vi "Dashboard Main.vi"() -> ()   [LabVIEW 2015]
uses:
  Common Code/Auton Command Cluster.ctl
  Common Code/Auton File Lists.ctl
  Vision/Camera Types.ctl
  Common Code/Goal Vision Packet.ctl
  <vilib>/Rock Robotics/WPI/Camera/WPI_CameraSettings Read MJPG.ctl
  <vilib>/Rock Robotics/WPI/Camera/WPI_CameraImageSize.ctl
  Common Code/Encoder Values Super Cluster.ctl
  Common Code/Encoder Values.ctl
  Common Code/Power and Diagnostic Data.ctl
  Common Code/Utilities/PDP Data.ctl
  Common Code/Utilities/PCM Data.ctl
  Common Code/IMU Data.ctl
  navX-MXP Library/COMMON/TypeDefs/Value TypeDefs/navX NAVX_CAL_STATUS.ctl
  navX-MXP Library/COMMON/TypeDefs/Value TypeDefs/navX NAVX_OP_STATUS.ctl
  Common Code/Intake Status Cluster.ctl
  Common Code/Intake Mode.ctl
  Common Code/Intake States.ctl
  Common Code/Climb Status Cluster.ctl
  Common Code/Climb Presets.ctl
  Common Code/Major Loop Times.ctl
  Common Code/Shooter State Cluster.ctl
  Common Code/Shooter State.ctl
  Common Code/Shoot Modes Enum.ctl
  Common Code/Shot Type.ctl
  Common Code/Encoder Control.ctl
  Common Code/Drivetrain Status Cluster.ctl
  Common Code/Drivetrain Modes.ctl
  Common Code/Dist Drive Status.ctl
  Common Code/Drivetrain Settings.ctl
  Common Code/Shooter Presets.ctl
  Common Code/Shot Presets.ctl
  Common Code/Intake Presets.ctl
  Common Code/Drivetrain Output Range.ctl
  Common Code/Ultrasonic Data.ctl
  Common Code/Dashboard Communication/Dashboard Control Data.ctl
  Common Code/Dashboard Drivetrain Command.ctl
  Common Code/Drivetrain Vision.ctl
  Common Code/Ball Tracking Command Cluster.ctl
  Common Code/Ball Vision Packet.ctl
  Common Code/Tracking Mode.ctl
  Common Code/IntakeEcoderControl.ctl
  Common Code/Dashboard Communication/Dashboard Display Data.ctl
  <vilib>/Rock Robotics/WPI/Dashboard/WPI_DashboardLogging Global.vi
  <vilib>/Utility/inputDevices.llb/keyboardAcquire.vi
  navX-MXP Library/navX-MXP IMU.lvlib
panel:
  in  "Logging Filename":path=path ""
  in  "stop":bool
  out "DumbDashMessage":string="111 values loaded OK"
  in  "Save":bool
  in  "Load":bool
  in  "TCP":refnum<k5>
  in  "Rec Mode":enum32{"Stop", "Record", "Playback"}(radio)
  out "Image Message":string="Timeout in Camera Communications"
  in  "Dashboard Tab":T1(tab)=enum."Shoot"
  out "Intake State":bool
  out "Right RPM":dbl(knob) scale=0.0..5000.0
  out "Left RPM":dbl(knob) scale=0.0..5000.0
  out "Mode":T2(ring)=enum."Disconnected"
  out "Shooter Mode":bool
  out "Gyro":dbl(knob) scale=0.0..360.0 scale format="%#.7g"
  out "Climb Mode":bool
  out "Intake Mode":bool
  out "Shooter State":bool
  out "Camera IP":string
  out "Robot IP":string
  out "Angle Ready?":bool
  out "RPM Ready?":bool
  out "Vision Ready?":bool
  out "Ball Loaded?":bool
  out "Intake High?":bool
  out "Shooter Ready?":bool
  out "Front Camera Display":T3(plugin-control)
  in  "Camera Mode":u16(ring)=3 items=["Camera Off", "USB Camera SW", "USB Camera HW", "IP Camera"]
  out "FPS":dbl
  out "Bandwidth (Mbps)":dbl
  out "NAVX_CAL_STATUS":T4 items=["IMU_CAL_STATE_MASK"=3, "IMU_CAL_INPROGRESS"=0, "IMU_CAL_ACCUMULATE"=1, "IMU_CAL_COMPLETE"=2, "MAG_CAL_COMPLETE"=4, "BARO_CAL_COMPLETE"=8]
  out "Auton Command Cluster":T5
  out "Auton File Lists":T6
  in  "Ultrasonic Limit":dbl
  in  "Roll Limit":dbl
  in  "Pitch Limit":dbl
  in  "Drivetrain Settings":T7={"Gyro Tolerance"=6.0, "Throttle Ramp (ms)"=250.0, "Angular rate compensation"=FALSE, "Throttle to Rate Scale"=0.0, "Rate compensation gain"=0.0, "Kv"=0.0, "Ka"=0.0, "Feed Forward P"=1.0, "Feed Forward D"=0.0, "Goal Vision PID gains"={"proportional gain (Kc)"=0.0, "integral time (Ti, min)"=0.0, "derivative time (Td, min)"=0.0}, "Goal Detection Window"=0.1} {"Goal Vision PID gains"."derivative time (Td, min)" format="%.3f"; "Goal Vision PID gains"."integral time (Ti, min)" format="%.3f"; "Goal Vision PID gains"."proportional gain (Kc)" format="%.3f"}
  out "Drivetrain Status Cluster":T8 {"2nd Gear Time" scale=0.0..135.0; "1st Gear Time" scale=0.0..135.0}
  in  "Encoder Settings":T11={"Right Tick Constant"=0.002781, "Left Tick Constant"=0.002785, "Reset?"=FALSE, "Y Dist"={"PID gains"={"proportional gain (Kc)"=0.0, "integral time (Ti, min)"=0.0, "derivative time (Td, min)"=0.0}}, "Y Stop Thresh"=0.0, "Y Stop Speed"=0.0}
  in  "Goal Output Range":cluster{"output high":dbl, "output low":dbl}
  out "Encoder Values":T12
  in  "Steer PID output":cluster{"output high":dbl, "output low":dbl}
  in  "Steer PID gains":T14
  in  "Shooter Presets":T15={"Batter Shot"={"Left Wheel RPM"=0.0, "Right Wheel RPM"=0.0, "Angle"=0.0}, "Deep Middle Shot"={"Left Wheel RPM"=0.0, "Right Wheel RPM"=0.0, "Angle"=0.0}, "Manual Shot"={"Left Wheel RPM"=700.0, "Right Wheel RPM"=700.0, "Angle"=0.0}, "Left Ticks Per Rotation"=-1378.0, "Right Ticks Per Rotation"=1388.0, "Low Bar Shot"={"Left Wheel RPM"=0.0, "Right Wheel RPM"=0.0, "Angle"=0.0}, "Shooter RPM Tolerance"=50.0, "IIR Filter Power"=0.0, "Trigger Power"=0.9, "Fire from Load Delay"=250, "Angle Pot M"=12.0, "Angle Pot B"=-0.1, "Shooter Length"=0.0, "String Pot Dist"=0.0, "Angle PID gains"={"proportional gain (Kc)"=1.0, "integral time (Ti, min)"=0.0, "derivative time (Td, min)"=0.002}, "Angle Motor Output"={"output high"=0.0, "output low"=0.0}, "Shooter Angle Tolerance"=3.0, "Vision Shoot x^2"=0.0, "Vision Shoot x"=0.0, "Dist from Axis Cam to Pivot"=23.375, "High Goal Center Height"=97.0, "Feed Forward Max Accel"=0.0, "Feed Forward Kv"=0.005, "Backwards Trigger"=-0.4, "Shot Finish Delay (ms)"=250.0, "Angle Max Current"=40.0, "Angle Current Trip Time"=500.0, "Shooter Intake Angle"=0.0, "Vision Shoot c"=0.0, "Reset?"=FALSE, "Servo Release Delay"=0.0, "Servo Idle Angle"=108, "Servo Hold Angle"=55, "Angle Pot x^2"=0.0, "Angle Pot x"=0.0, "Angle Pot c"=0.0, "Ignore Angle?"=FALSE} {"Angle Motor Output"."output low" format="%.2f"; "Angle Motor Output"."output high" format="%.2f"}
  out "Shooter State Cluster":T17 {"Trigger Output" scale=-1.0..1.0; "Angle Motor Output" scale=-1.0..1.0; "Right RPM" scale=0.0..5000.0; "Left RPM" scale=0.0..5000.0}
  in  "Intake Presets":T21={"Intake Speed"=0.8, "Outake Speed"=-0.8, "Low Height"=0.0, "Half Height"=55.0, "Full Height"=90.0, "Angle Speed"=0.0, "Fast Angle"=0.0, "Encoder Scale"=0.001478, "Load Height"=30.0, "Output Range"={"output high"=0.0, "output low"=0.0}, "Rotation Power Max/Min"=0.5, "MaxCurrent"=40.0, "Intake Trip Time"=500.0, "Idle Height"=40.0, "Max Height"=90.0, "Reset Encoders?"=FALSE, "PID gains"={"proportional gain (Kc)"=1.0, "integral time (Ti, min)"=0.0, "derivative time (Td, min)"=0.0}} {"Max Height" format="%#_7g"; "Idle Height" format="%#_7g"; "Intake Trip Time" format="%#_7g"; "MaxCurrent" format="%#_7g"; "Rotation Power Max/Min" format="%#_7g"; "Load Height" format="%#_7g"; "Encoder Scale" format="%#_7g"; "Fast Angle" format="%#_7g"; "Angle Speed" format="%#_7g"; "Full Height" format="%#_7g"; "Half Height" format="%#_7g"; "Low Height" format="%#_7g"; "Outake Speed" format="%#_7g"; "Intake Speed" format="%#_7g"}
  out "Intake Status Cluster":T23
  in  "Climb Presets":T26
  out "Climb Status Cluster":T27
  out "IMU Data":T28 {"NAVX_OP_STATUS" items=["INITIALIZING", "SELFTEST_IN_PROGRESS", "ERROR", "IMU_AUTOCAL_IN_PROGRESS", "NORMAL"]; "NAVX_CAL_STATUS" items=["IMU_CAL_STATE_MASK"=3, "IMU_CAL_INPROGRESS"=0, "IMU_CAL_ACCUMULATE"=1, "IMU_CAL_COMPLETE"=2, "MAG_CAL_COMPLETE"=4, "BARO_CAL_COMPLETE"=8]}
  out "Gyro 2":dbl(knob) scale=0.0..360.0 scale format="%#.7g"
  out "Ultrasonic Data":T30
  out "Camera Display 2":T3(plugin-control)
  in  "Aspect Fudge Factor":dbl=1.0
  in  "Score Threshold 2":dbl=75.0 format="%#_13g"
  out "Goal Display":T3(plugin-control)
  out "Found Targets":T31(array[cluster]) {"Normalized Rect"."Numeric 5" format="%#_2g"; "Normalized Rect"."Numeric 3" format="%#_2g"; "Normalized Rect"."Numeric 2" format="%#_2g"; "Normalized Rect"."Numeric" format="%#_2g"}
  in  "Camera Type":T32=enum."1011"
  out "Goal Vision Packet":T33
  in  "Camera Settings 2":T34={"fps"=30, "compression"=30, "Image Size"=enum."320x240"}
  in  "File number":i32
  in  "Use Goal File?":bool
  in  "Color Components":T36={"Hue"={110.0, 142.0}, "Sat"={138.0, 255.0}, "Val"={139.0, 198.0}} {"Val" scale=0.0..255.0; "Sat" scale=0.0..255.0; "Hue" scale=0.0..255.0 scale format="%#_3g"}
  out "Goal Active?":bool
  out "Power and Diagnostic Data":T37
  out "Control Info":T40
  out "Status Info":T41
  out "DS TCP":T42
  out "Robot Metrics":T43
  out "Loop Times":T44
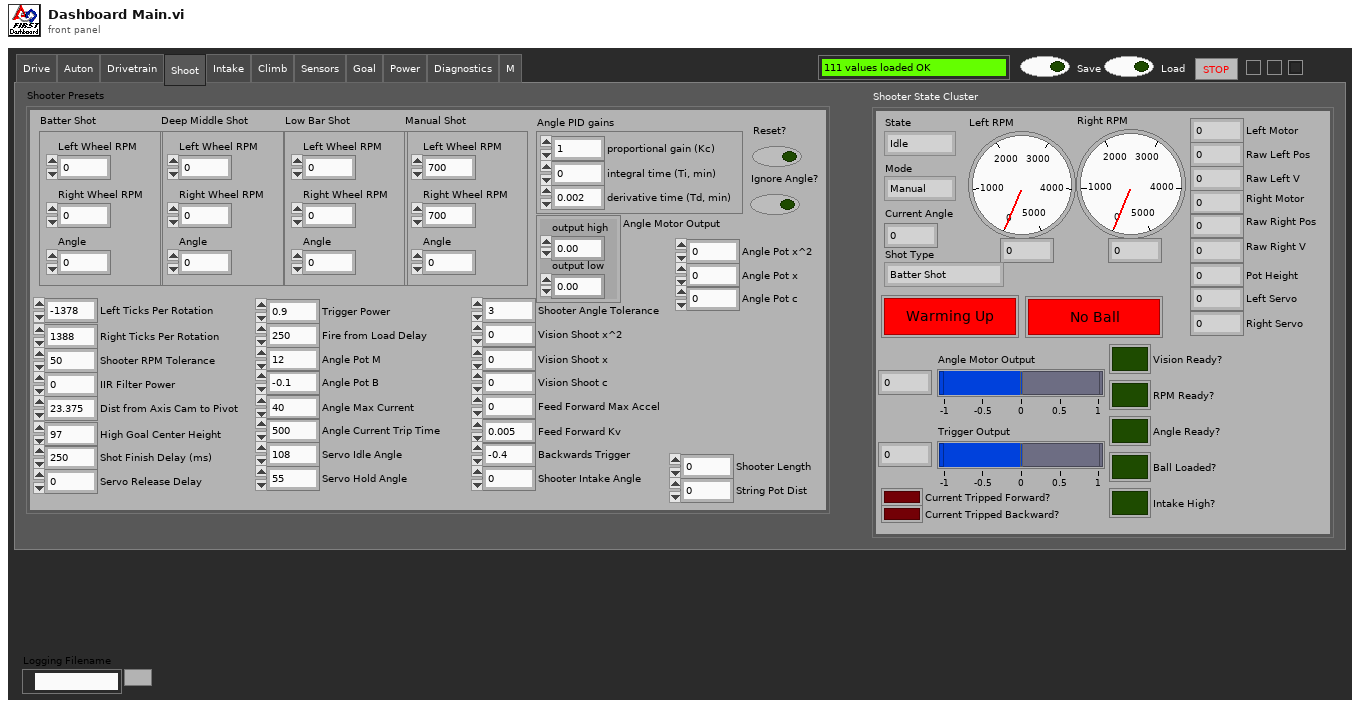
[diagram p1: front panel]
types:
  T1 = enum32{"Drive", "Auton", "Drivetrain", "Shoot", "Intake", "Climb", "Sensors", "Goal", "Power", "Diagnostics", "M"}
  T2 = enum8{"Tele-Op Disabled", "Tele-Op Enabled", "Auto Disabled", "Auto Enabled", "Test Disabled", "Test Enabled", "Disconnected", "No Code", "E-Stop"}
  T3 = typedef "IMAQ Image.ctl" = refnum<image>
  T4 = typedef "navX-MXP IMU.lvlib/navX NAVX_CAL_STATUS.ctl" = u8
  T5 = typedef "Auton Command Cluster.ctl" = cluster{"Command ID":i32, "maxTime":dbl, "Y Distance":dbl, "Heading":dbl, "Throttle":dbl, "Async":dbl, "Velocity":dbl, "Acceleration":dbl, "To":dbl, "Condition":dbl, "Shot Type":dbl, "Left RPM":dbl, "Override RPM":i32, "Override Angle":i32, "Right RPM":dbl, "Angle":dbl, "Intake Mode":i32, "Intake Cmd":i32, "Intake O":i32, "Eject O":i32, "Angle O":i32, "Arm O":i32, "Intake Speed":dbl, "Eject Speed":dbl, "Arm Angle":dbl, "Arm Speed":dbl, "Intake?":i32, "Eject?":i32}
  T6 = typedef "Auton File Lists.ctl" = cluster{"Current Queue":string, "General Scripts":string, "Defense Scripts":string, "Movement Scripts":string}
  T7 = typedef "Drivetrain Settings.ctl" = cluster{"Gyro Tolerance":dbl, "Throttle Ramp (ms)":dbl, "Angular rate compensation":bool, "Throttle to Rate Scale":dbl, "Rate compensation gain":dbl, "Kv":dbl, "Ka":dbl, "Feed Forward P":dbl, "Feed Forward D":dbl, "Goal Vision PID gains":cluster{"proportional gain (Kc)":dbl, "integral time (Ti, min)":dbl, "derivative time (Td, min)":dbl}, "Goal Detection Window":dbl}
  T8 = typedef "Drivetrain Status Cluster.ctl" = cluster{"Modes":T9, "Y (Throttle)":dbl, "X (Steer)":dbl, "Gyro In Range?":bool, "Distance Drive Finished?":bool, "Stop Eject Lockout":bool, "Dist Drive Status":T10, "Y Target":dbl, "Heading Target":dbl, "Vision Target Aligned?":bool, "Gear":dbl, "1st Gear Time":dbl, "2nd Gear Time":dbl, "1st Gear Shifts":dbl, "2nd Gear Shifts":dbl}
  T9 = typedef "Drivetrain Modes.ctl" = enum16{"Climb", "Manual", "Ball Vision Targeting", "Goal Vision Targeting", "PID Distance Drive", "Hybrid"}
  T10 = typedef "Dist Drive Status.ctl" = cluster{"Y In Range":bool, "X In Range":bool, "Gyro In Range":bool, "Y Dist":dbl, "X Dist":dbl, "Gyro":dbl}
  T11 = typedef "Encoder Control.ctl" = cluster{"Right Tick Constant":dbl, "Left Tick Constant":dbl, "Reset?":bool, "Y Dist":cluster{"PID gains":cluster{"proportional gain (Kc)":dbl, "integral time (Ti, min)":dbl, "derivative time (Td, min)":dbl}}, "Y Stop Thresh":dbl, "Y Stop Speed":dbl}
  T12 = typedef "Encoder Values Super Cluster.ctl" = cluster{"Left Encoder":T13, "Right Encoder":T13}
  T13 = typedef "Encoder Values.ctl" = cluster{"Distance":dbl, "Speed":dbl, "Ticks":dbl}
  T14 = cluster{"proportional gain (Kc)":dbl, "integral time (Ti, min)":dbl, "derivative time (Td, min)":dbl}
  T15 = typedef "Shooter Presets.ctl" = cluster{"Batter Shot":T16, "Deep Middle Shot":T16, "Manual Shot":T16, "Left Ticks Per Rotation":dbl, "Right Ticks Per Rotation":dbl, "Low Bar Shot":T16, "Shooter RPM Tolerance":dbl, "IIR Filter Power":dbl, "Trigger Power":dbl, "Fire from Load Delay":i32, "Angle Pot M":dbl, "Angle Pot B":dbl, "Shooter Length":dbl, "String Pot Dist":dbl, "Angle PID gains":cluster{"proportional gain (Kc)":dbl, "integral time (Ti, min)":dbl, "derivative time (Td, min)":dbl}, "Angle Motor Output":cluster{"output high":dbl, "output low":dbl}, "Shooter Angle Tolerance":dbl, "Vision Shoot x^2":dbl, "Vision Shoot x":dbl, "Dist from Axis Cam to Pivot":dbl, "High Goal Center Height":dbl, "Feed Forward Max Accel":dbl, "Feed Forward Kv":dbl, "Backwards Trigger":dbl, "Shot Finish Delay (ms)":dbl, "Angle Max Current":dbl, "Angle Current Trip Time":dbl, "Shooter Intake Angle":dbl, "Vision Shoot c":dbl, "Reset?":bool, "Servo Release Delay":dbl, "Servo Idle Angle":i32, "Servo Hold Angle":i32, "Angle Pot x^2":dbl, "Angle Pot x":dbl, "Angle Pot c":dbl, "Ignore Angle?":bool}
  T16 = typedef "Shot Presets.ctl" = cluster{"Left Wheel RPM":dbl, "Right Wheel RPM":dbl, "Angle":dbl}
  T17 = typedef "Shooter State Cluster.ctl" = cluster{"State":T18, "Left RPM":dbl, "Right RPM":dbl, "Shooter Ready?":bool, "Ball Loaded?":bool, "Current Angle":dbl, "Angle Motor Output":dbl, "Trigger Output":dbl, "Angle Ready?":bool, "RPM Ready?":bool, "Vision Ready?":bool, "Ball Loaded?":bool, "Mode":T19, "Shot Type":T20, "Pot Height":dbl, "Current Tripped Forward?":bool, "Current Tripped Backward?":bool, "Left Motor":dbl, "Right Motor":dbl, "Intake High?":bool, "Raw Left Pos":dbl, "Raw Right Pos":dbl, "Raw Left V":dbl, "Raw Right V":dbl, "Right Servo":i32, "Left Servo":i32}
  T18 = typedef "Shooter State.ctl" = enum16{"Idle", "Warmup", "Shooter Ready", "Shoot"}
  T19 = typedef "Shoot Modes Enum.ctl" = enum16{"Manual", "Safe", "Auto"}
  T20 = typedef "Shot Type.ctl" = enum16{"Batter Shot", "Corner Shot", "Curve Shot", "Vision Shot", "Deep Middle Shot"}
  T21 = typedef "Intake Presets.ctl" = cluster{"Intake Speed":dbl, "Outake Speed":dbl, "Low Height":dbl, "Half Height":dbl, "Full Height":dbl, "Angle Speed":dbl, "Fast Angle":dbl, "Encoder Scale":dbl, "Load Height":dbl, "Output Range":T22, "Rotation Power Max/Min":dbl, "MaxCurrent":dbl, "Intake Trip Time":dbl, "Idle Height":dbl, "Max Height":dbl, "Reset Encoders?":bool, "PID gains":cluster{"proportional gain (Kc)":dbl, "integral time (Ti, min)":dbl, "derivative time (Td, min)":dbl}}
  T22 = typedef "Drivetrain Output Range.ctl" = cluster{"output high":dbl, "output low":dbl}
  T23 = typedef "Intake Status Cluster.ctl" = cluster{"Roller Power":dbl, "Angle Power":dbl, "Intake Mode":T24, "Intake States":T25, "Rollers Active?":bool, "Current Height":dbl, "Target Height":dbl, "Encoder Raw Position":dbl, "Forward Tripped?":bool, "Backward Tripped?":bool, "Override IR?":bool}
  T24 = typedef "Intake Mode.ctl" = enum16{"Safe", "Auto", "Manual"}
  T25 = typedef "Intake States.ctl" = enum16{"Idle", "Set roller speed", "Move to angle"}
  T26 = typedef "Climb Presets.ctl" = cluster{"Pull Power":dbl, "Unpin Power":dbl, "Time to Hold":dbl}
  T27 = typedef "Climb Status Cluster.ctl" = cluster{"Pull Power":dbl, "Unpin Power":dbl, "PTO Engaged?":bool, "Pull Height":dbl}
  T28 = typedef "IMU Data.ctl" = cluster{"Pitch":sgl, "Roll":sgl, "Yaw":sgl, "Data Valid?":bool, "Temp":sgl, "MOVING":bool, "YAW_STABLE":bool, "Accel X":sgl, "Accel Y":sgl, "Accel Z":sgl, "Accel Magnitude":sgl, "Pitch Rate":sgl, "Roll Rate":sgl, "Yaw Rate":sgl, "NavX Opened?":bool, "NAVX_CAL_STATUS":T4, "NAVX_OP_STATUS":T29}
  T29 = typedef "navX-MXP IMU.lvlib/navX NAVX_OP_STATUS.ctl" = u8
  T30 = typedef "Ultrasonic Data.ctl" = cluster{"Left Ultrasonic":dbl, "Right Ultrasonic":dbl}
  T31 = cluster{"Distance (ft)":dbl, "Center":cluster{dbl, dbl}, "Normalized Rect":cluster{"Numeric":dbl, "Numeric 2":dbl, "Numeric 3":dbl, "Numeric 5":dbl}}[]
  T32 = typedef "Camera Types.ctl" = enum16{"206", "1011", "1013", "MS HD3000 square", "MS HD3000 640x480"}
  T33 = typedef "Goal Vision Packet.ctl" = cluster{"Distance":dbl, "Center X":dbl, "Center Y":dbl, "Found Target?":bool}
  T34 = typedef "WPI_CameraSettings Read MJPG.ctl" = cluster{"fps":i32, "compression":i32, "Image Size":T35}
  T35 = typedef "WPI_CameraImageSize.ctl" = enum16{"640x480", "320x240", "160x120", "Custom"}
  T36 = cluster{"Hue":cluster{dbl, dbl}, "Sat":cluster{dbl, dbl}, "Val":cluster{dbl, dbl}}
  T37 = typedef "Power and Diagnostic Data.ctl" = cluster{"PDP Data":T38, "PCM Data":T39, "roboRIO input voltage (V)":dbl, "roboRIO input current (A)":dbl, "3.3V Rail Short":bool, "5 V Rail Short":bool, "6 V Rail Short":bool, "roboRIO Brownout":bool, "Outputs Enabled?":bool}
  T38 = typedef "PDP Data.ctl" = cluster{"Battery Voltage":sgl, "Temperature (degrees C)":sgl, "Internal Battery R (Ohms)":sgl, "Energy (J)":sgl, "Power (W)":sgl, "Total Current (A)":sgl, "Battery Voltage Fault":bool, "Temperature Fault":bool, "Hardware Fault":bool, "Currents":cluster{"[0]":sgl, "[1]":sgl, "[2]":sgl, "[3]":sgl, "[4]":sgl, "[5]":sgl, "[6]":sgl, "[7]":sgl, "[8]":sgl, "[9]":sgl, "[10]":sgl, "[11]":sgl, "[12]":sgl, "[13]":sgl, "[14]":sgl, "[15]":sgl}, "Current Faults":cluster{"[0]":bool, "[1]":bool, "[2]":bool, "[3]":bool, "[4]":bool, "[5]":bool, "[6]":bool, "[7]":bool, "[8]":bool, "[9]":bool, "[10]":bool, "[11]":bool, "[12]":bool, "[13]":bool, "[14]":bool, "[15]":bool}}
  T39 = typedef "PCM Data.ctl" = cluster{"Compressor Fault":bool, "Solenoid Fault":bool, "Compressor Enabled":bool, "Hardware Fault":bool, "Compressor Current":dbl}
  T40 = cluster{"Control Bits":cluster{"TestMode":bool, "Autonomous":bool, "Enabled":bool, "FMS Present":bool, bool, bool, bool, "E-Stop":bool}, "Team Station ":u8, "Countdown":sgl, "Joystick Values":cluster{"Axes":dbl[], "Buttons":bool[], "POVs":i16[]}[]}
  T41 = cluster{"Status bits":cluster{"Test Mode":bool, "Autonomous":bool, "Enabled":bool, "Code Start":bool, "Brownout":bool, "Reserved 2":bool, "Reserved 3":bool, "E-Stop":bool}, "Code Trace":cluster{"Disabled":bool, "TeleOp":bool, "Auto":bool, "Test":bool}, "Controller Type":enum16{"unknown", "cRIO", "roboRio"}, "Code?":enum16{"unknown", "noCode", "code"}, "Battery V":dbl}
  T42 = cluster{"Error Strings":string, "Disable Counts":cluster{u16, u16}, "Rail Faults":cluster{u16, u16, u16}, "Robot IP":string, "DB Mode":u8, "Event Info":cluster{"Name":string, "Type":u8, "Number":u16, "Replay":u8}, "Camera Addr":string}
  T43 = cluster{"Storage":cluster{"Disk Free":u64, "RAM Block":u32, "RAM free":u32}, "CPU Utilization":cluster{"CPU % ISR":sgl, "CPU % Time Crit":sgl, "CPU % Timed Str":sgl, "CPU % High":sgl, "CPU % Above":sgl, "CPU % Normal":sgl, "CPU % Low":sgl}, "CAN":cluster{"% Bus Utilization":sgl, "Bus Off Cnt":u32, "TX_FIFO Full Cnt":u32, "Receive Error Cnt":u8, "Transmit Error Cnt":u8}, "HID":cluster{"HID Outputs":u32, "Rumble Low":u16, "Rumble High":u16}[]}
  T44 = typedef "Major Loop Times.ctl" = cluster{"DT Loop Timer":u32, "Shooter Loop Timer":u32, "Intake Loop Timer":u32, "US Loop Timer":u32, "Auton File Loop Timer":u32}
  T45 = typedef "Image Type" = u32
  T46 = cluster{cluster{dbl, dbl}, cluster{dbl, dbl}, cluster{dbl, dbl}}
  T47 = cluster{"Score":sgl, "Fitted Circle":cluster{"Center":cluster{"X":sgl, "Y":sgl}, "Radius":dbl, "Circle Rect":cluster{"L":sgl, "T":sgl, "R":sgl, "B":sgl}, "Roundness":dbl, "SNR (dB)":dbl}, "Search Rect":cluster{"L":sgl, "T":sgl, "R":sgl, "B":sgl}, "Details":cluster{"Edge":sgl, "Area":sgl, "Circ":sgl, "Diam":sgl}}[]
  T48 = typedef "Ball Tracking Command Cluster.ctl" = cluster{"Distance to Ball":dbl, "Desired Angle":dbl, "Command":enum16{"Turn to Ball", "Turn to Angle", "Get Distance"}, "Pixels from Center":dbl}
  T49 = typedef "Tracking Mode.ctl" = enum16{"Turn to Ball", "Turn to Angle"}
  T50 = enum16{"Turn to Ball", "Turn to Angle", "Get Distance"}
  T51 = typedef "NI_LVConfig.lvlib/Config Data RefNum.ctl" = refnum<k1>
  T52 = cluster{"Bounding box":cluster{"left":dbl, "top":dbl, "right":dbl, "bottom":dbl}, "Aspect Ratio":dbl, "Area to CH":dbl, "X Mask":dbl, "Y Mask":dbl, "Moment":dbl}[]
  T53 = cluster{"Distance (ft)":dbl, "Center":cluster{dbl, dbl}, "Normalized Rect":cluster{"Numeric":dbl, "Numeric 2":dbl, "Numeric 3":dbl, "Numeric 5":dbl}}
  T54 = typedef "Dashboard Display Data.ctl" = cluster{"Auton Command Cluster":T5, "Auton File Lists":T6, "Drivetrain Status Cluster":T8, "Encoder Values":T12, "IMU Data":T28, "Power and Diagnostic Data":T37, "Gyro":dbl, "Shooter State Cluster":T17, "Intake Status Cluster":T23, "Ultrasonic Data":T30, "Climb Status Cluster":T27, "Loop Times":T44}
  T55 = typedef "Dashboard Control Data.ctl" = cluster{"Shooter Presets":T15, "Encoder Control":T11, "Steer PID output":cluster{"output high":dbl, "output low":dbl}, " Steer PID gains":cluster{"proportional gain (Kc)":dbl, "integral time (Ti, min)":dbl, "derivative time (Td, min)":dbl}, "Drivetrain Settings":T7, "Vision Packet":T33, "Dashboard Drivetrain Command":T56, "Info/Command Cluster":T48, "Ball Vision Packet":T58, "Intake Presets":T21, "Intake Encoder Control":T59, "Climb Presets":T26, "Ultrasonic Limit":dbl, "Roll Limit":dbl, "Pitch Limit":dbl, "Goal Output Range":cluster{"output high":dbl, "output low":dbl}}
  T56 = typedef "Dashboard Drivetrain Command.ctl" = cluster{"Drivetrain Vision":T57}
  T57 = typedef "Drivetrain Vision.ctl" = cluster{"Goal Window":dbl, "Ball Window":dbl}
  T58 = typedef "Ball Vision Packet.ctl" = cluster{"Ball Detected?":bool, "Distance to Ball":dbl, "Desired Angle":dbl, "Pixels from Center":dbl, "Tracking mode":T49}
  T59 = typedef "IntakeEcoderControl.ctl" = cluster{"Arm Tick Constant":dbl, "Reset?":bool, "Y Dist":cluster{"PID gains":cluster{"proportional gain (Kc)":dbl, "integral time (Ti, min)":dbl, "derivative time (Td, min)":dbl}}, "Y Stop Thresh":dbl, "Y Stop Speed":dbl}
  T60 = cluster{"Image Size":bool, "Image Type":bool, "Pixel Value":bool, "ROI Information":bool, "Zoom Factor":bool}
  T61 = enum16{"0", "1", "2", "3", "4", "5", "6", "7", "8", "9", "A", "B", "C", "D", "E", "F", "G", "H", "I", "J", "K", "L", "M", "N", "O", "P", "Q", "R", "S", "T", "U", "V", "W", "X", "Y", "Z", "F1", "F2", "F3", "F4", "F5", "F6", "F7", "F8", "F9", "F10", "F11", "F12", "F13", "F14", "F15", "ADD", "BACK", "BACKSLASH", "CAPITAL", "COMMA", "DECIMAL", "DELETE", "DIVIDE", "DOWN", "END", "EQUALS", "ESCAPE", "GRAVE (`)", "HOME", "INSERT", "LBRACKET", "LCONTROL", "LEFT", "L ALT", "LSHIFT", "LWIN", "MINUS", "MULTIPLY", "NEXT", "NUMLOCK", "NUMPAD_0", "NUMPAD_1", "NUMPAD_2", "NUMPAD_3", "NUMPAD_4", "NUMPAD_5", "NUMPAD_6", "NUMPAD_7", "NUMPAD_8", "NUMPAD_9", "PAUSE", "PERIOD", "PRIOR (PG UP)", "RBRACKET", "RCONTROL", "RETURN", "RIGHT", "R ALT", "RSHIFT", "RWIN", "SCROLL", "SEMICOLON", "SLASH", "SPACE", "SUBTRACT", "TAB", "UP", "ENTER (num pad)", "' (quote)"}[]
  T62 = typedef "DumbDash Control.ctl" = cluster{"Name":string, "Ref":refnum<vi>, "Type":T63}
  T63 = typedef "DumbDash Control Type.ctl" = enum16{"Invalid", "Number", "Boolean", "String"}
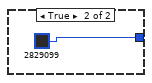
[diagram p2: hidden frame]
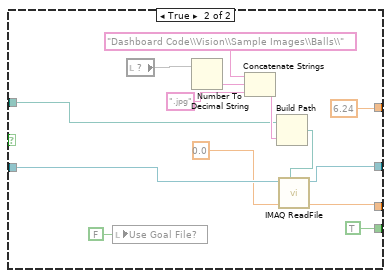
[diagram p3: hidden frame]
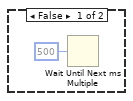
[diagram p4: hidden frame]
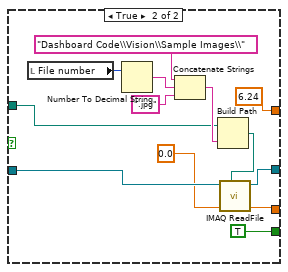
[diagram p6: hidden frame]
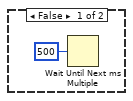
[diagram p7: hidden frame]
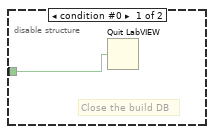
[diagram p9: hidden frame]
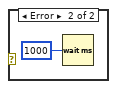
[diagram p12: hidden frame]
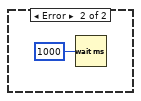
[diagram p13: hidden frame]
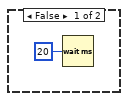
[diagram p14: hidden frame]
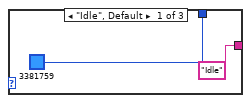
[diagram p15: hidden frame]
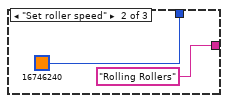
[diagram p16: hidden frame]
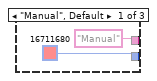
[diagram p17: hidden frame]
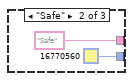
[diagram p18: hidden frame]
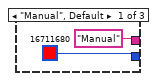
[diagram p20: hidden frame]
diagram:
  w3 = T45 0 items=["Grayscale (U8)", "Grayscale (I16)", "Grayscale (SGL)", "Complex (CSG)", "RGB (U32)", "HSL (U32)", "RGB (U64)", "Grayscale (U16)"] ("Image Type")
  w8 = T45 4 items=["Grayscale (U8)", "Grayscale (I16)", "Grayscale (SGL)", "Complex (CSG)", "RGB (U32)", "HSL (U32)", "RGB (U64)", "Grayscale (U16)"] ("Image Type")
  w11 = enum16{"Stop", "Record", "Playback"}."Stop"
  w17 = 1340
  w18 = 500
  w22 = enum32{"Stop", "Record", "Playback"}."Stop" ("Rec Mode")
  (unwired) "This VI has seven parallel loops for different tasks and a bit of initialization code that runs just once.\n\nTypical dashboard extensions only need to edit the panel. Adding new indicators or controls simply involves placing them on the panel in the Operations tab and naming them the same as the SmartDashboard variable on the robot\n\nIf the display needs to process the data before display, loop one is an example of doing that for the joysticks and motors.\n\nIf you want customize the video display or perform processing on it, loop two is where that takes place.\n\nOther loops should not need to be modified. They are pretty standard, and document the task they perform."  # Documentation
  # "Command Param Info"
  # "Started one, Unique ID holds\nresponse"
  # "Loop 7. Wait for DS connections"
  # "Basic debug and auto controls: Their data names are fixed, but\nthe displayed name, called a caption, can be changed directly or in\nrobot code such as shown in Begin."
  # "Controls for Test Mode, Camera Settings, etc."
  # "Additional UI Initialization"
  # "Loop 6. Animation for background of window during playback and record"
  # "Fires each time robot IP\nchanges, simulator does this"
  # "Fires each time window\ndocking changes."
  # "Collects all controls and indicators\nin the Basic and Custom tab.\nIf you need to bind additional controls,\nadd their references. You can extend the\nenum constant or use an integer."
  # "The remaining code below this line typically doesn't need to be modified."
  # "Loop 4. Process UI events related to test mode, checklist, and camera settings"
  # "Terminals of controls and indicators that are bound to the smart dashboard by name.\nYou can place the terminals anywhere you like and even read data from them.\nYou bind controls by adding the control reference to the array on the left. The subVI will\ndo this for the contents of a tab, and you can do it for individual items too, as shown with\nthe LED. To create get the reference, right-click and Create>>Reference."
  # "Loop 5. Adjusts placement onscreen, hides the titlebar, etc."
  # "Loop 1. Receive various data streams from Driver Station, update joystick, motors, and more complex displays that don't easily bind to variables."
  n1 = control-ref of="Rec Mode"() -> ()  [unwired: 1 out]
  n2 = control-ref of="Dashboard Tab"() -> ()  [unwired: 1 out]
  n3 = Obtain Notifier(name (unnamed)="Robot IP Update", notification data type="IP Addr" ("name (unnamed)")) -> (notifier out=w16:refnum<notifier>)  [unwired: 2 in, 2 out]
  n4 = property class="VI" props=["Front Panel.Closeable"]() -> (reference out=w21:refnum<vi>)  [unwired: 2 in, 2 out]
  n5 = Obtain Notifier(name (unnamed)="Window Mode", notification data type=TRUE) -> (notifier out=w20:refnum<notifier>)  [unwired: 2 in, 2 out]
  n6 = disable-structure shown="Disabled" {
    frame Disabled {
      w41 = T45 0 items=["Grayscale (U8)", "Grayscale (I16)", "Grayscale (SGL)", "Complex (CSG)", "RGB (U32)", "HSL (U32)", "RGB (U64)", "Grayscale (U16)"] ("Image Type")
      w43 = T45 4 items=["Grayscale (U8)", "Grayscale (I16)", "Grayscale (SGL)", "Complex (CSG)", "RGB (U32)", "HSL (U32)", "RGB (U64)", "Grayscale (U16)"] ("Image Type")
      n7 = call <vilib>:"Application Directory.vi"() -> ("Application Directory"=w40:path)
      n8 = call "IMAQ Create"("Image Name"="Ball Detection", "Image Type"=w43) -> ("New Image"=w39:T3, "error out"=w38:errorcluster)  [unwired: 3 in]
      n9 = call "IMAQ Create"("Image Name"="Ball Mask", "Image Type"=w41) -> ("New Image"=w37:T3, "error out"=w36:errorcluster)  [unwired: 3 in]
      n10 = while {
        tunnel: w38 -> [_]
        tunnel: w37 -> [w48]
        tunnel: w36 -> [_]
        tunnel: w39 -> [w52]
        tunnel: w40 -> [w53]
        stop <- FALSE stop-if-true
        n11 = case shown="False" w47 {
          tunnel: [w60 TRUE ("Active")] -> w50
          tunnel: w52 -> [w61 w75]
          tunnel: [w59 w74] -> w49
          tunnel: w53 -> [_ w70]
          tunnel: [w57 6.24 ("Bandwidth (Mbps)")] -> w46
          tunnel: [w58 0.0 ("FPS")] -> w51
          frame False {
            n12 = local read "Rec Mode"() -> (w62:enum32{"Stop", "Record", "Playback"})
            n13 = call "624WPI_CameraRead MJPG for Dashboard.vi"("Rec Mode"=w62, "Camera IP"="10.6.24.23", "Refnum in"=w61) -> ("Active"=w60:bool, "Refnum out"=w59:T3, "FPS"=w58:dbl, "Bandwidth (Mbps)"=w57:dbl, "Camera Settings"=w54:T34, "Camera Mode"=w55:u16)  [unwired: 3 in]
          }
          frame True {
            n14 = local write "Use Goal File?"(FALSE ("Use Goal File?")) -> ()
            n15 = local read item#-1() -> (w66)
            n16 = Number To Decimal String(number=w66) -> (decimal integer string=w73:string)  [unwired: 1 in]
            n17 = Concatenate Strings("Dashboard Code\\Vision\\Sample Images\\Balls\\", w73, ".jpg" ("string")) -> (w71:string)
            n18 = Build Path(base path=w70, name or relative path=w71) -> (appended path=w69:path)
            n19 = call "IMAQ ReadFile"("File Path"=w69, "Image"=w75) -> ("Image Out"=w74:T3)  [unwired: 5 in, 4 out]
          }
        }
        n20 = case shown="True" w50 {
          tunnel: w51 -> [_ w95]
          tunnel: w46 -> [_ w96]
          tunnel: w49 -> [_ w101]
          tunnel: w48 -> [_ w98]
          frame False {
            n21 = Wait Until Next ms Multiple(millisecond multiple=u32 500) -> ()  [unwired: 1 out]
          }
          frame True {
            w102 = u16 2 items=["RGB", "HSL", "HSV", "HSI", "CIE L*a*b*", "CIE XYZ"] ("Color Mode")
            n22 = call "IMAQ Clear Overlay"("Image"=w101) -> ("Image Out"=w89:T3)  [unwired: 9 in, 1 out]
            n23 = local read item#-1() -> (w90)
            n24 = local read item#-1() -> (w94)
            n25 = call "Calibration Helper2.vi"("Color Mode"=w102, "Color Components"=w94, "Image"=w89) -> ("Changed"=w100:bool, "output color"=w99:T46, "Image Ctl Refnum"=w93:refnum<vi>)  [unwired: 6 in]
            n26 = Select(t=w99, s=w100, f=w94) -> (s? t:f=w97:T46)
            n27 = call "Find Balls.vi"("Color Components"=w97, "Score Cutoff"=w90, "Image Dst."=w98, "Image Src."=w89) -> ("Ranked Objects"=w85:T47, "Annotated Image"=w92:T3, "Initial Image"=w91:T3)  [unwired: 4 in, 1 out]
            n28 = local read item#-1() -> (w88)
            n29 = local write item#-1(w97) -> ()
            n30 = Array Size(array=w85) -> (size(s)=w84:i32)
            n31 = call "Track Best Ball.vi"("Ball Camera Type"=w88, "Camera Image"=w89, "Ranked Balls"=w85) -> ("Ball Track Cluster"=w86:T48, "Tracking mode"=w87:T49)  [unwired: 7 in]
            n32 = Not Equal To 0?(x=w84) -> (x != 0?=w81:bool)
            n33 = Unbundle By Name(w86) -> ("Distance to Ball"=w80:dbl, "Desired Angle"=w79:dbl, "Command"=w77:T50, "Pixels from Center"=w78:dbl)
            n34 = local read item#-1() -> (w82)
            n35 = Bundle By Name(cluster=w82, "Tracking mode"=w77, "Desired Angle"=w79, "Distance to Ball"=w80, "Pixels from Center"=w78, "Ball Detected?"=w81) -> (w83:cluster{})
          }
        }
      }
    }
    frame Enabled {
    }
  }
  n36 = call "624WPIAdjust Dashboard Window.vi"("Width"=w17, "Height"=w18, "VI"=w21, "Notifier in"=w20) -> ()  [unwired: 8 in]
  n37 = call "IMAQ Create"("Image Name"="Goal Detection", "Image Type"=w8) -> ("New Image"=w10:T3, "error out"=w9:errorcluster)  [unwired: 3 in]
  n38 = vi-ref "Playback Controls.vi"() -> (w26:refnum<vi>)
  n39 = call "IMAQ Create"("Image Name"="Goal Mask", "Image Type"=w3) -> ("New Image"=w6:T3, "error out"=w5:errorcluster)  [unwired: 3 in]
  n40 = call "Initialize Camera and CheckList.vi"() -> ("Array"=w31:cluster{string[]}[], "File Refnum"=w30:T51)  [unwired: 9 in, 1 out]
  n41 = call <vilib>:"Application Directory.vi"() -> ("Application Directory"=w2:path)
  n42 = call "624WPIAdjust Dashboard Window.vi"("Width"=w17, "Height"=w18, "VI"=w21, "Notifier in"=w20) -> ()  [unwired: 8 in]
  n43 = register-events(refnum<vi> refnum) -> (reference out=w25:refnum<event-registration>, error out=w24:errorcluster)  [unwired: 2 in]
  n44 = while {
    tunnel: w9 -> [_]
    tunnel: w6 -> [w111]
    tunnel: w5 -> [_]
    tunnel: w10 -> [w109]
    tunnel: w2 -> [w107]
    stop <- FALSE stop-if-true
    n45 = case shown="False" "Use Goal File?" {
      tunnel: [w115 TRUE] -> w110
      tunnel: w109 -> [w120 w131]
      tunnel: [w114 w130] -> w108
      tunnel: w107 -> [_ w125]
      tunnel: [w112 6.24 ("Bandwidth (Mbps)")] -> w105
      tunnel: [w113 0.0 ("FPS")] -> w104
      frame False {
        n46 = local read "Rec Mode"() -> (w117:enum32{"Stop", "Record", "Playback"})
        n47 = call "624WPI_CameraRead MJPG for Dashboard.vi"("Camera Settings"="Camera Settings 2", "Rec Mode"=w117, "Camera IP"="axis-camera.local", "Camera Mode"="Camera Mode", "Refnum in"=w120) -> ("Active"=w115:bool, "Refnum out"=w114:T3, "FPS"=w113:dbl, "Bandwidth (Mbps)"=w112:dbl)  [unwired: 3 in]
      }
      frame True {
        n48 = local read "File number"() -> (w123:i32)
        n49 = Number To Decimal String(number=w123) -> (decimal integer string=w128:string)  [unwired: 1 in]
        n50 = Concatenate Strings("Dashboard Code\\Vision\\Sample Images\\", w128, ".jpg" ("string")) -> (w126:string)
        n51 = Build Path(base path=w125, name or relative path=w126) -> (appended path=w124:path)
        n52 = call "IMAQ ReadFile"("File Path"=w124, "Image"=w131) -> ("Image Out"=w130:T3)  [unwired: 5 in, 4 out]
      }
    }
    "Goal Active?" <- w110
    n53 = case shown="True" w110 {
      tunnel: w108 -> [_ w172]
      tunnel: w111 -> [_ w148]
      tunnel: w105 -> [_ w158]
      tunnel: w104 -> [_ w157]
      frame False {
        n54 = Wait Until Next ms Multiple(millisecond multiple=u32 500) -> ()  [unwired: 1 out]
      }
      frame True {
        w138 = 2 ("y")
        w151 = u16 2 items=["RGB", "HSL", "HSV", "HSI", "CIE L*a*b*", "CIE XYZ"] ("Color Mode")
        n55 = local read "Color Components"() -> (w152:T36)
        n56 = call "IMAQ Clear Overlay"("Image"=w172) -> ("Image Out"=w156:T3)  [unwired: 9 in, 1 out]
        n57 = control-ref of="Camera Display 2"() -> (w155:refnum<vi>)
        n58 = local read "Score Threshold 2"() -> (w173:dbl)
        n59 = local read "Camera Type"() -> (w169:T32)
        n60 = call "Calibration Helper2.vi"("Color Mode"=w151, "Color Components"=w152, "Image"=w156, "Image Ctl Refnum"=w155) -> ("Changed"=w154:bool, "output color"=w153:T46)  [unwired: 6 in]
        n61 = Select(t=w153, s=w154, f=w152) -> (s? t:f=w150:T36)
        n62 = local write "Color Components"(w150) -> ()
        n63 = call "Find Goals.vi"("Aspect Fudge Factor"="Aspect Fudge Factor", "Score Threshold"=w173, "Color"=w150, "Image Dst"=w148, "Image Src"=w156) -> ("Targets"=w171:T52, "Masked Image"=w170:T3)  [unwired: 5 in]
        n64 = call "Track Goal.vi"("Original Image"=w156, "Camera Type"=w169, "Targets"=w171, "Goal Display"=w170) -> ("Target Line Masking Out"=w134:T3, "Best Target Available"=w168:T53, "Found Targets"=w160:T31, "Goal Display"=→"Goal Display":T3)  [unwired: 4 in]
        "Found Targets" <- w160
        "Camera Display 2" <- w134
        n65 = Array Size(array=w160) -> (size(s)=w161:i32)
        n66 = Unbundle By Name(w168) -> ("Distance (ft)"=w166:dbl, "Center"=w165:cluster{dbl, dbl})
        n67 = Not Equal To 0?(x=w161) -> (x != 0?=w159:bool)
        n68 = Unbundle(w165) -> (w164:dbl, w163:dbl)
        n69 = Bundle By Name(cluster=T33 {"Distance"=0.0, "Center X"=0.0, "Center Y"=0.0, "Found Target?"=FALSE}, "Distance"=w166, "Center X"=w164, "Center Y"=w163, "Found Target?"=w159) -> (→"Goal Vision Packet":T33)
        n70 = call "IMAQ GetImageSize"("Image"=w134) -> ("Y Resolution"=w136:i32, "X Resolution"=w139:i32)  [unwired: 3 in, 1 out]
        n71 = Divide(x=w139, y=w138) -> (x/y=w144:dbl)
        n72 = Divide(x=w139, y=w138) -> (x/y=w142:dbl)
        n73 = Bundle(cluster=cluster{"X":i32, "Y":i32} {"X"=0, "Y"=0} ("Start Point"), "X"=w144, "Y"=0) -> (w140:cluster{"X":i32, "Y":i32})
        n74 = Bundle(cluster=cluster{"X":i32, "Y":i32} {"X"=0, "Y"=0} ("Start Point"), "X"=w142, "Y"=w136) -> (w137:cluster{"X":i32, "Y":i32})
        n75 = call "IMAQ Overlay Line"("Color"=u32 6618880, "End Point"=w137, "Start Point"=w140, "Image"=w134) -> ("Image Out"=→"Front Camera Display":T3)  [unwired: 6 in, 1 out]
        "Bandwidth (Mbps)" <- w158
        "FPS" <- w157
      }
    }
  }
  n76 = property class="VI"() -> ("Panel"=w28:refnum<vi>)  [unwired: 2 in, 2 out]
  n77 = while {
    tunnel: [w184] -> _
    tunnel: w16 -> [w183]
    tunnel: w20 -> [w181]
    i -> [w184]
    stop <- FALSE stop-if-true
    n78 = call "624WPI_DashboardGetInfo.vi"("Binding Refnum"=w183, "Window Mode Notifier"=w181, "TCP Cnx"="TCP") -> ("Power and Errors"=w180:T42, "Robot Metrics"=w179:T43, "Status Info"=w178:T41, "Control Info"=w177:T40, "Robot Mode"=w176:T2, "Process?"=w175:bool, "Custom Dashboard Data"=w174:string)  [unwired: 2 in]
    "Mode" <- w176
    n79 = case shown="True" w175 {
      tunnel: w178 -> [_ w235]
      tunnel: w179 -> [_ w234]
      tunnel: w177 -> [_ w236]
      tunnel: w180 -> [_ w233]
      tunnel: w176 -> [_ _]
      tunnel: w174 -> [_ w230]
      frame False {
        n80 = Wait (ms)(milliseconds to wait=u32 20) -> ()  [unwired: 1 out]
      }
      frame True {
        n81 = Unbundle By Name(w233) -> ("Robot IP"=→"Robot IP":string, "Camera Addr"=→"Camera IP":string)
        n82 = Unflatten From String(type=T54 {"Auton Command Cluster"={"Command ID"=0, "maxTime"=0.0, "Y Distance"=0.0, "Heading"=0.0, "Throttle"=0.0, "Async"=0.0, "Velocity"=0.0, "Acceleration"=0.0, "To"=0.0, "Condition"=0.0, "Shot Type"=0.0, "Left RPM"=0.0, "Override RPM"=0, "Override Angle"=0, "Right RPM"=0.0, "Angle"=0.0, "Intake Mode"=0, "Intake Cmd"=0, "Intake O"=0, "Eject O"=0, "Angle O"=0, "Arm O"=0, "Intake Speed"=0.0, "Eject Speed"=0.0, "Arm Angle"=0.0, "Arm Speed"=0.0, "Intake?"=0, "Eject?"=0}, "Auton File Lists"={"Current Queue"="", "General Scripts"="", "Defense Scripts"="", "Movement Scripts"=""}, "Drivetrain Status Cluster"={"Modes"=enum."Manual", "Y (Throttle)"=0.0, "X (Steer)"=0.0, "Gyro In Range?"=FALSE, "Distance Drive Finished?"=FALSE, "Stop Eject Lockout"=FALSE, "Dist Drive Status"={"Y In Range"=FALSE, "X In Range"=FALSE, "Gyro In Range"=FALSE, "Y Dist"=0.0, "X Dist"=0.0, "Gyro"=0.0}, "Y Target"=0.0, "Heading Target"=0.0, "Vision Target Aligned?"=FALSE, "Gear"=0.0, "1st Gear Time"=0.0, "2nd Gear Time"=0.0, "1st Gear Shifts"=0.0, "2nd Gear Shifts"=0.0}, "Encoder Values"={"Left Encoder"={"Distance"=0.0, "Speed"=0.0, "Ticks"=0.0}, "Right Encoder"={"Distance"=0.0, "Speed"=0.0, "Ticks"=0.0}}, "IMU Data"={"Pitch"=0.0, "Roll"=0.0, "Yaw"=0.0, "Data Valid?"=FALSE, "Temp"=0.0, "MOVING"=FALSE, "YAW_STABLE"=FALSE, "Accel X"=0.0, "Accel Y"=0.0, "Accel Z"=0.0, "Accel Magnitude"=0.0, "Pitch Rate"=0.0, "Roll Rate"=0.0, "Yaw Rate"=0.0, "NavX Opened?"=FALSE, "NAVX_CAL_STATUS"=0, "NAVX_OP_STATUS"=0}, "Power and Diagnostic Data"={"PDP Data"={"Battery Voltage"=0.0, "Temperature (degrees C)"=0.0, "Internal Battery R (Ohms)"=0.0, "Energy (J)"=0.0, "Power (W)"=0.0, "Total Current (A)"=0.0, "Battery Voltage Fault"=FALSE, "Temperature Fault"=FALSE, "Hardware Fault"=FALSE, "Currents"={"[0]"=0.0, "[1]"=0.0, "[2]"=0.0, "[3]"=0.0, "[4]"=0.0, "[5]"=0.0, "[6]"=0.0, "[7]"=0.0, "[8]"=0.0, "[9]"=0.0, "[10]"=0.0, "[11]"=0.0, "[12]"=0.0, "[13]"=0.0, "[14]"=0.0, "[15]"=0.0}, "Current Faults"={"[0]"=FALSE, "[1]"=FALSE, "[2]"=FALSE, "[3]"=FALSE, "[4]"=FALSE, "[5]"=FALSE, "[6]"=FALSE, "[7]"=FALSE, "[8]"=FALSE, "[9]"=FALSE, "[10]"=FALSE, "[11]"=FALSE, "[12]"=FALSE, "[13]"=FALSE, "[14]"=FALSE, "[15]"=FALSE}}, "PCM Data"={"Compressor Fault"=FALSE, "Solenoid Fault"=FALSE, "Compressor Enabled"=FALSE, "Hardware Fault"=FALSE, "Compressor Current"=0.0}, "roboRIO input voltage (V)"=0.0, "roboRIO input current (A)"=0.0, "3.3V Rail Short"=FALSE, "5 V Rail Short"=FALSE, "6 V Rail Short"=FALSE, "roboRIO Brownout"=FALSE, "Outputs Enabled?"=FALSE}, "Gyro"=0.0, "Shooter State Cluster"={"State"=enum."Idle", "Left RPM"=0.0, "Right RPM"=0.0, "Shooter Ready?"=FALSE, "Ball Loaded?"=FALSE, "Current Angle"=0.0, "Angle Motor Output"=0.0, "Trigger Output"=0.0, "Angle Ready?"=FALSE, "RPM Ready?"=FALSE, "Vision Ready?"=FALSE, "Ball Loaded?"=FALSE, "Mode"=enum."Manual", "Shot Type"=enum."Batter Shot", "Pot Height"=0.0, "Current Tripped Forward?"=FALSE, "Current Tripped Backward?"=FALSE, "Left Motor"=0.0, "Right Motor"=0.0, "Intake High?"=FALSE, "Raw Left Pos"=0.0, "Raw Right Pos"=0.0, "Raw Left V"=0.0, "Raw Right V"=0.0, "Right Servo"=0, "Left Servo"=0}, "Intake Status Cluster"={"Roller Power"=0.0, "Angle Power"=0.0, "Intake Mode"=enum."Auto", "Intake States"=enum."Idle", "Rollers Active?"=FALSE, "Current Height"=0.0, "Target Height"=0.0, "Encoder Raw Position"=0.0, "Forward Tripped?"=FALSE, "Backward Tripped?"=FALSE, "Override IR?"=FALSE}, "Ultrasonic Data"={"Left Ultrasonic"=0.0, "Right Ultrasonic"=0.0}, "Climb Status Cluster"={"Pull Power"=0.0, "Unpin Power"=0.0, "PTO Engaged?"=FALSE, "Pull Height"=0.0}, "Loop Times"={"DT Loop Timer"=0, "Shooter Loop Timer"=0, "Intake Loop Timer"=0, "US Loop Timer"=0, "Auton File Loop Timer"=0}}, binary string=w230) -> (value=w214:T54)  [unwired: 3 in, 2 out]
        n83 = Unbundle By Name(w214) -> ("Auton Command Cluster"=→"Auton Command Cluster":T5, "Auton File Lists"=→"Auton File Lists":T6, "Shooter State Cluster"=w205:T17, "Encoder Values"=→"Encoder Values":T12, "Drivetrain Status Cluster"=→"Drivetrain Status Cluster":T8, "IMU Data"=w197:T28, "Power and Diagnostic Data"=→"Power and Diagnostic Data":T37, "Gyro"=→"Gyro" →"Gyro 2":dbl, "Intake Status Cluster"=w213:T23, "Climb Status Cluster"=→"Climb Status Cluster":T27, "Loop Times"=→"Loop Times":T44, "Ultrasonic Data"=→"Ultrasonic Data":T30)
        "IMU Data" <- w197
        "Intake Status Cluster" <- w213
        "Shooter State Cluster" <- w205
        n84 = Unbundle By Name(w205) -> ("Right RPM"=→"Right RPM":dbl, "Left RPM"=→"Left RPM":dbl, "Angle Ready?"=→"Angle Ready?":bool, "RPM Ready?"=→"RPM Ready?":bool, "Vision Ready?"=→"Vision Ready?":bool, "Ball Loaded?"=→"Ball Loaded?":bool, "Intake High?"=→"Intake High?":bool, "Shooter Ready?"=→"Shooter Ready?":bool, "State"=w224:T18, "Mode"=w223:T19)
        n85 = disable-structure shown="Disabled" {
          frame Disabled {
            n86 = Unbundle By Name() -> ("Intake Mode"=w245:T24)  [unwired: 1 in]
            n87 = case shown="\"Auto\"" w245 {
              tunnel: ["Manual" "Safe" "Auto"] -> w247
              tunnel: [u32 16711680 u32 16770560 u32 6618880] -> w244
              frame "Manual", Default {
              }
              frame "Safe" {
              }
              frame "Auto" {
              }
            }
            n88 = Bundle(w244, w244) -> (w243:cluster{u32, u32})  [unwired: 1 in]
            n89 = Build Array(w243) -> (w246:cluster{u32, u32}[])
            n90 = property on="Intake Mode" class="Bool (strict)"("BoolText.Text"=w247, "Colors [4]"=w246) -> ()  [unwired: 2 in, 2 out]
          }
          frame Enabled {
          }
        }
        n91 = Unbundle By Name(w213) -> ("Intake States"=w192:T25, "Intake Mode"=w210:T24)
        n92 = Unbundle By Name(w197) -> ("NAVX_CAL_STATUS"=→"NAVX_CAL_STATUS":T4)
        n93 = case shown="\"Shooter Ready\"" w224 {
          tunnel: ["Idle" "Warmup" "Shooter Ready" "Shooting"] -> w219
          tunnel: [u32 3381759 u32 16746240 u32 16711680 u32 6618880] -> w222
          frame "Idle", Default {
          }
          frame "Warmup" {
          }
          frame "Shooter Ready" {
          }
          frame "Shoot" {
          }
        }
        n94 = case shown="\"Manual\", Default" w223 {
          tunnel: ["Manual" "Safe" "Auto"] -> w227
          tunnel: [u32 16711680 u32 16770560 u32 6618880] -> w228
          frame "Manual", Default {
          }
          frame "Safe" {
          }
          frame "Auto" {
          }
        }
        n95 = case shown="\"Auto\"" w210 {
          tunnel: ["Manual" "Safe" "Auto"] -> w208
          tunnel: [u32 16711680 u32 16770560 u32 6618880] -> w211
          frame "Manual", Default {
          }
          frame "Safe" {
          }
          frame "Auto" {
          }
        }
        n96 = case shown="\"Move to angle\"" w192 {
          tunnel: ["Idle" "Rolling Rollers" "Moving to Angle"] -> w196
          tunnel: [u32 3381759 u32 16746240 u32 16711680] -> w195
          frame "Idle", Default {
          }
          frame "Set roller speed" {
          }
          frame "Move to angle" {
          }
        }
        n97 = Bundle(w228, w228) -> (w225:cluster{u32, u32})  [unwired: 1 in]
        n98 = Build Array(w225) -> (w226:cluster{u32, u32}[])
        n99 = Bundle(w211, w211) -> (w212:cluster{u32, u32})  [unwired: 1 in]
        n100 = Bundle(w222, w222) -> (w221:cluster{u32, u32})  [unwired: 1 in]
        n101 = property on="Shooter Mode" class="Bool (strict)"("BoolText.Text"=w227, "Colors [4]"=w226) -> ()  [unwired: 2 in, 2 out]
        n102 = Build Array(w212) -> (w209:cluster{u32, u32}[])
        n103 = Build Array(w221) -> (w220:cluster{u32, u32}[])
        n104 = property on="Intake Mode" class="Bool (strict)"("BoolText.Text"=w208, "Colors [4]"=w209) -> ()  [unwired: 2 in, 2 out]
        n105 = property on="Shooter State" class="Bool (strict)"("BoolText.Text"=w219, "Colors [4]"=w220) -> ()  [unwired: 2 in, 2 out]
        n106 = Bundle(w195, w195) -> (w194:cluster{u32, u32})  [unwired: 1 in]
        n107 = Build Array(w194) -> (w193:cluster{u32, u32}[])
        n108 = property on="Intake State" class="Bool (strict)"("Colors [4]"=w193, "BoolText.Text"=w196) -> ()  [unwired: 2 in, 2 out]
        "Control Info" <- w236
        "Status Info" <- w235
        "Robot Metrics" <- w234
        "DS TCP" <- w233
      }
    }
  }
  n109 = while {
    stop <- FALSE stop-if-true
    n110 = local read "Goal Vision Packet"() -> (w282:T33)
    n111 = Bundle By Name(cluster=T55 {"Shooter Presets"={"Batter Shot"={"Left Wheel RPM"=0.0, "Right Wheel RPM"=0.0, "Angle"=0.0}, "Deep Middle Shot"={"Left Wheel RPM"=0.0, "Right Wheel RPM"=0.0, "Angle"=0.0}, "Manual Shot"={"Left Wheel RPM"=0.0, "Right Wheel RPM"=0.0, "Angle"=0.0}, "Left Ticks Per Rotation"=0.0, "Right Ticks Per Rotation"=0.0, "Low Bar Shot"={"Left Wheel RPM"=0.0, "Right Wheel RPM"=0.0, "Angle"=0.0}, "Shooter RPM Tolerance"=0.0, "IIR Filter Power"=0.0, "Trigger Power"=0.0, "Fire from Load Delay"=0, "Angle Pot M"=0.0, "Angle Pot B"=0.0, "Shooter Length"=0.0, "String Pot Dist"=0.0, "Angle PID gains"={"proportional gain (Kc)"=1.0, "integral time (Ti, min)"=0.01, "derivative time (Td, min)"=0.0}, "Angle Motor Output"={"output high"=0.0, "output low"=0.0}, "Shooter Angle Tolerance"=0.0, "Vision Shoot x^2"=0.0, "Vision Shoot x"=0.0, "Dist from Axis Cam to Pivot"=0.0, "High Goal Center Height"=97.0, "Feed Forward Max Accel"=0.0, "Feed Forward Kv"=0.0, "Backwards Trigger"=0.0, "Shot Finish Delay (ms)"=0.0, "Angle Max Current"=0.0, "Angle Current Trip Time"=0.0, "Shooter Intake Angle"=0.0, "Vision Shoot c"=0.0, "Reset?"=FALSE, "Servo Release Delay"=0.0, "Servo Idle Angle"=0, "Servo Hold Angle"=0, "Angle Pot x^2"=0.0, "Angle Pot x"=0.0, "Angle Pot c"=0.0, "Ignore Angle?"=FALSE}, "Encoder Control"={"Right Tick Constant"=0.0, "Left Tick Constant"=0.0, "Reset?"=FALSE, "Y Dist"={"PID gains"={"proportional gain (Kc)"=0.0, "integral time (Ti, min)"=0.0, "derivative time (Td, min)"=0.0}}, "Y Stop Thresh"=0.0, "Y Stop Speed"=0.0}, "Steer PID output"={"output high"=0.0, "output low"=0.0}, " Steer PID gains"={"proportional gain (Kc)"=0.0, "integral time (Ti, min)"=0.0, "derivative time (Td, min)"=0.0}, "Drivetrain Settings"={"Gyro Tolerance"=0.0, "Throttle Ramp (ms)"=0.0, "Angular rate compensation"=FALSE, "Throttle to Rate Scale"=1.0, "Rate compensation gain"=0.01, "Kv"=0.0, "Ka"=0.0, "Feed Forward P"=0.0, "Feed Forward D"=0.0, "Goal Vision PID gains"={"proportional gain (Kc)"=1.0, "integral time (Ti, min)"=0.01, "derivative time (Td, min)"=0.0}, "Goal Detection Window"=0.0}, "Vision Packet"={"Distance"=0.0, "Center X"=0.0, "Center Y"=0.0, "Found Target?"=FALSE}, "Dashboard Drivetrain Command"={"Drivetrain Vision"={"Goal Window"=0.0, "Ball Window"=0.0}}, "Info/Command Cluster"={"Distance to Ball"=0.0, "Desired Angle"=0.0, "Command"=enum."Turn to Ball", "Pixels from Center"=0.0}, "Ball Vision Packet"={"Ball Detected?"=FALSE, "Distance to Ball"=0.0, "Desired Angle"=0.0, "Pixels from Center"=0.0, "Tracking mode"=enum."Turn to Ball"}, "Intake Presets"={"Intake Speed"=0.0, "Outake Speed"=0.0, "Low Height"=0.0, "Half Height"=0.0, "Full Height"=0.0, "Angle Speed"=0.0, "Fast Angle"=0.0, "Encoder Scale"=0.0, "Load Height"=0.0, "Output Range"={"output high"=0.0, "output low"=0.0}, "Rotation Power Max/Min"=0.0, "MaxCurrent"=0.0, "Intake Trip Time"=0.0, "Idle Height"=0.0, "Max Height"=0.0, "Reset Encoders?"=FALSE, "PID gains"={"proportional gain (Kc)"=0.0, "integral time (Ti, min)"=0.0, "derivative time (Td, min)"=0.0}}, "Intake Encoder Control"={"Arm Tick Constant"=0.0, "Reset?"=FALSE, "Y Dist"={"PID gains"={"proportional gain (Kc)"=0.0, "integral time (Ti, min)"=0.0, "derivative time (Td, min)"=0.0}}, "Y Stop Thresh"=0.0, "Y Stop Speed"=0.0}, "Climb Presets"={"Pull Power"=0.0, "Unpin Power"=0.0, "Time to Hold"=0.0}, "Ultrasonic Limit"=0.0, "Roll Limit"=0.0, "Pitch Limit"=0.0, "Goal Output Range"={"output high"=0.0, "output low"=0.0}} ("anything"), "Shooter Presets"="Shooter Presets", "Goal Output Range"="Goal Output Range", "Vision Packet"=w282, "Drivetrain Settings"="Drivetrain Settings", "Steer PID output"="Steer PID output", "Steer PID gains"="Steer PID gains", "Intake Presets"="Intake Presets", "Climb Presets"="Climb Presets", "Encoder Control"="Encoder Settings", "Ultrasonic Limit"="Ultrasonic Limit", "Roll Limit"="Roll Limit", "Pitch Limit"="Pitch Limit") -> (w287:T55)
    n112 = Flatten To String(anything=w287) -> (data string=w289:string)  [unwired: 3 in, 2 out]
    n113 = Wait (ms)(milliseconds to wait=u32 250) -> ()  [unwired: 1 out]
    n114 = local read "Robot IP"() -> (w291:string)
    n115 = call "DumbDash Send.vi"("Robot IP"=w291, "data string"=w289) -> ()  [unwired: 10 in]
  }
  n116 = while {
    tunnel: w31 -> [w300]
    shift-right: [w292] -> _
    shift-left: w30 -> [w299]
    tunnel: [w298] -> _
    tunnel: w26 -> [w297]
    tunnel: w25 -> [w296]
    tunnel: w24 -> [_]
    tunnel: w21 -> [w295]
    shift-right: [w293] -> _
    shift-left: _ -> [w294]
    i -> [w298]
    stop <- FALSE stop-if-true
    n117 = event shown="[0] \"Rec Mode\": Value Change" {
      selector: w296 -> [_ _ _]
      dyn-events: [w304 _ _] -> _
      timeout: _ -> [_ _ _]
      tunnel: w300 -> [_ _ _]
      tunnel: w299 -> [w309 _ _]
      tunnel: w297 -> [w308 _ w322]
      tunnel: w295 -> [w307 _ _]
      tunnel: w294 -> [_ _ _]
      tunnel: [0 _ _] -> w293
      tunnel: [w309 _ _] -> w292
      event "Rec Mode": Value Change {
        n118 = event-data() -> ("NewVal"=w302:enum32{"Stop", "Record", "Playback"})  [unwired: 1 in]
        n119 = case shown="\"Playback\"" w302 {
          tunnel: w308 -> [_ w312 w316]
          tunnel: [_ _ w320] -> w304
          tunnel: [_ _ w319] -> _
          tunnel: w307 -> [_ _ w314]
          tunnel: cluster{i32, i32} {-250, 170} -> [_ _ w313]
          tunnel: [_ _ T60 {"Image Size"=TRUE, "Image Type"=TRUE, "Pixel Value"=TRUE, "ROI Information"=TRUE, "Zoom Factor"=FALSE} ("Image Information Shown:All Elements")] -> _
          tunnel: [_ _ TRUE ("Zoom Factor")] -> _
          frame Default {
          }
          frame "Stop", "Record" {
            # "Place Window too"
            n120 = invoke class="VI" method="FP.Close"(reference=w312) -> (reference out=w311:refnum<vi>)  [unwired: 2 in, 2 out]
            n121 = invoke class="VI" method="Abort VI"(reference=w311) -> ()  [unwired: 2 in, 3 out]
          }
          frame "Playback" {
            n122 = call "Open Playback Panel.vi"("Offset"=w313, "DB VI Ref"=w314, "Playback in"=w316) -> ("Playback out"=w315:refnum<vi>)  [unwired: 8 in]
            n123 = register-events(w315) -> (reference out=w320:refnum<event-registration>, error out=w319:errorcluster)  [unwired: 2 in]
          }
        }
        n124 = global write "WPI_DashboardLogging Global.vi" "Logging Filename"(path "") -> ()
        n125 = global write "WPI_DashboardLogging Global.vi" "Recording"(w302) -> ()
        n126 = call <vilib>:"WPI_DashboardNT Log FieldName Cache.vi"("Operation"=enum16{"Lookup/Add", "Index", "Clear"}."Clear") -> ()  [unwired: 8 in, 3 out]
      }
      event Panel Close {
        w321 = enum32{"Stop", "Record", "Playback"}."Stop" ("Rec Mode")
        n127 = event-data() -> ()  [unwired: 1 in, 4 out]
        n128 = local write "Rec Mode"(w321) -> ()
        n129 = global write "WPI_DashboardLogging Global.vi" "Recording"(w321) -> ()
      }
      event Panel Close {
        n130 = event-data() -> ()  [unwired: 1 in, 4 out]
        n131 = invoke class="VI" method="FP.Close"(reference=w322) -> (reference out=w324:refnum<vi>)  [unwired: 2 in, 2 out]
        n132 = invoke class="VI" method="Abort VI"(reference=w324) -> (error out=w323:errorcluster)  [unwired: 2 in, 2 out]
        n133 = invoke class="VI" method="Abort VI"(error in=w323) -> ()  [unwired: 2 in, 3 out]
      }
    }
  }
  n134 = property class="Pnl"(reference=w28) -> ("Panes[]"=w29:refnum<vi>[])  [unwired: 1 in, 2 out]
  n135 = Index Array(array=w29) -> (element=w27:refnum<vi>)  [unwired: 1 in]
  n136 = while {
    tunnel: w27 -> [w326]
    i -> [w329]
    stop <- FALSE stop-if-true
    n137 = Wait (ms)(milliseconds to wait=u32 100) -> ()  [unwired: 1 out]
    n138 = case shown="\"Record\"" "Rec Mode" {
      tunnel: w329 -> [_ _ w344]
      tunnel: [u32 2829099 ("Base Color") u32 11141120 ("Target Color") w333] -> w325
      frame "Stop", Default {
        # "Reset the color, extra updates don't cost much"
      }
      frame "Record" {
      }
      frame "Playback" {
        # "Playback"
        n139 = Quotient & Remainder(x=w344, y=u32 50 ("milliseconds to wait")) -> (x-y*floor(x/y)=w340:u32)  [unwired: 1 out]
        n140 = Divide(x=w340, y=u32 50 ("milliseconds to wait")) -> (x/y=w337:dbl)
        n141 = Multiply(x=6.283185307179586, y=w337) -> (x*y=w342:dbl)
        n142 = Sine(x=w342) -> (sin(x)=w341:dbl)
        n143 = Absolute Value(x=w341) -> (abs(x)=w334:dbl)
        n144 = call "Interpolate RGB Color.vi"("Proportion"=w334, "Target Color"=u32 30976, "Base Color"=u32 2829099) -> ("Result Color"=w333:u32)  [unwired: 8 in]
      }
    }
    n145 = property class="Pane"(reference=w326, "PaneColor"=w325) -> ()  [unwired: 1 in, 2 out]
  }
  n146 = call <vilib>:"Intialize Keyboard.vi"() -> ("device ID"=w1:refnum<k1>)  [unwired: 10 in, 1 out]
  n147 = while {
    tunnel: w1 -> [w349]
    stop <- FALSE stop-if-true
    n148 = local read "Robot IP"() -> (w347:string)
    n149 = call-poly <vilib>:"Acquire Input Data.vi"("device ID"=w349) -> ("keys pressed"=w348:T61)  [unwired: 16 in, 2 out]
    n150 = call "Send Keyboard Data.vi"("Robot IP"=w347, "keys pressed"=w348) -> ()  [unwired: 10 in]
    n151 = Wait (ms)(milliseconds to wait=50) -> ()  [unwired: 1 out]
  }
  n152 = global write "WPI_DashboardLogging Global.vi" "Recording"(w11) -> ()
  n153 = local write "Rec Mode"(w11) -> ()
  n154 = while {
    stop <- FALSE stop-if-true
    n155 = local read "IMU Data"() -> (w361:T28)
    n156 = local read "Mode"() -> (w357:T2)
    n157 = Unbundle By Name(w361) -> ("Data Valid?"=w360:bool)
    n158 = Equal?(x=w357, y=T2."Disconnected") -> (x = y?=w354:bool)
    n159 = Equal?(x=w357, y=T2."No Code") -> (x = y?=w355:bool)
    n160 = Or(x=w354, y=w355) -> (x .or. y?=w356:bool)
    n161 = Or(x=w360, y=w356) -> (x .or. y?=w353:bool)
    n162 = case shown="False" w353 {
      tunnel: [w362 u32 2829099 ("Base Color")] -> w350
      frame False {
        n163 = Tick Count (ms)() -> (millisecond timer value=w363:u32)
        n164 = Quotient & Remainder(x=w363, y=u32 1000 ("milliseconds to wait")) -> (x-y*floor(x/y)=w370:u32)  [unwired: 1 out]
        n165 = Divide(x=w370, y=u32 1000 ("milliseconds to wait")) -> (x/y=w367:dbl)
        n166 = Multiply(x=6.283185307179586, y=w367) -> (x*y=w372:dbl)
        n167 = Sine(x=w372) -> (sin(x)=w371:dbl)
        n168 = Absolute Value(x=w371) -> (abs(x)=w366:dbl)
        n169 = call "Interpolate RGB Color.vi"("Proportion"=w366, "Target Color"=u32 16711680, "Base Color"=u32 2829099) -> ("Result Color"=w362:u32)  [unwired: 8 in]
      }
      frame True {
      }
    }
    n170 = property on="Gyro" class="Knob (strict)"("BGColor"=w350) -> ()  [unwired: 2 in, 2 out]
    n171 = property on="Gyro 2" class="Knob (strict)"("BGColor"=w350) -> ()  [unwired: 2 in, 2 out]
    n172 = Wait (ms)(milliseconds to wait=u32 50) -> ()  [unwired: 1 out]
  }
  n173 = control-ref of="Dashboard Tab"() -> (w12:refnum<vi>)
  n174 = while {
    tunnel: u16 1741 ("timeout ms (25000)") -> [w376]
    stop <- FALSE stop-if-true
    n175 = TCP Create Listener(10:w376) -> (0:w375:errorcluster, 3:w377:refnum<k5>)  [unwired: 4 in, 1 out]
    n176 = case shown="No Error" w375 {
      selector: w375 -> [w379 _]
      tunnel: w377 -> [w380 _]
      frame No Error {
        n177 = while {
          tunnel: w380 -> [w383]
          tunnel: w379 -> [w382]
          stop <- FALSE stop-if-true
          n178 = TCP Wait On Listener(8:w382, 11:w383) -> (0:w384:errorcluster, 4:w385:refnum<k5>)  [unwired: 2 in, 3 out]
          n179 = local write "TCP"(w385) -> ()
          n180 = case shown="No Error" w384 {
            frame No Error {
            }
            frame Error {
              n181 = Wait (ms)(milliseconds to wait=u32 1000) -> ()  [unwired: 1 out]
            }
          }
        }
      }
      frame Error {
        n182 = Wait (ms)(milliseconds to wait=u32 1000) -> ()  [unwired: 1 out]
      }
    }
  }
  n183 = global write "WPI_DashboardLogging Global.vi" "Recording"(w22) -> ()
  n184 = local write "Rec Mode"(w22) -> ()
  n185 = call "DumbDash Load Controls.vi"("TabControl in"=w12) -> ("Array"=w14:T62[])  [unwired: 10 in]
  n186 = disable-structure shown="Disabled" {
    frame Disabled {
      n187 = while {
        stop <- FALSE stop-if-true
        n188 = event shown="[0] Mouse Enter" {
          selector: _ -> [_]
          dyn-events: _ -> [_]
          timeout: _ -> [_]
          event Mouse Enter {
            n189 = event-data() -> ()  [unwired: 1 in, 4 out]
            n190 = flat-sequence {
              frame #0 {
                n191 = Wait (ms)(milliseconds to wait=u32 3000) -> ()  [unwired: 1 out]
              }
              frame #1 {
                w390 = u32 3552822
                w392 = u32 3552822
                n192 = property on="DumbDashMessage" class="Str"("Text.BG Color"=w392, "Text.BG Color"=w392, "Blinking"=FALSE) -> ()  [unwired: 2 in, 2 out]
                n193 = property on="DumbDashMessage" class="Str"("Text.BG Color"=w390, "Text.BG Color"=w390, "Blinking"=FALSE) -> ()  [unwired: 2 in, 2 out]
              }
            }
          }
        }
      }
    }
    frame Enabled {
    }
  }
  n194 = control-ref of="DumbDashMessage"() -> (w13:refnum<vi>)
  n195 = while {
    tunnel: w14 -> [w398]
    tunnel: w13 -> [w396]
    stop <- FALSE stop-if-true
    n196 = Wait (ms)(milliseconds to wait=u32 250) -> ()  [unwired: 1 out]
    n197 = disable-structure shown="RUN_TIME_ENGINE==False, Default" {
      disable-tunnel: "stop" -> [w401 w402]
      frame condition #0 {
        # "Close the build DB"
        n198 = Quit LabVIEW(quit? (T)=w401) -> ()
      }
      frame condition #1 (active) {
        n199 = Stop(stop? (T)=w402) -> ()
      }
    }
    n200 = case shown="True" "Save" {
      tunnel: w398 -> [_ w409]
      tunnel: w396 -> [_ w408]
      frame False {
      }
      frame True {
        n201 = flat-sequence {
          tunnel: w409 -> [w411]
          tunnel: w408 -> [w410]
          frame #0 {
            n202 = call "DumbDash Save Values.vi"("Message Box"=w410, "Controls In"=w411) -> ()  [unwired: 10 in]
          }
          frame #1 {
            n203 = local write "Save"(FALSE) -> ()
          }
        }
      }
    }
    n204 = case shown="True" "Load" {
      tunnel: w398 -> [_ w404]
      tunnel: w396 -> [_ w403]
      frame False {
      }
      frame True {
        n205 = flat-sequence {
          tunnel: w404 -> [w406]
          tunnel: w403 -> [w405]
          frame #0 {
            n206 = call "DumbDash Load Values.vi"("Message Box"=w405, "Controls In"=w406) -> ()  [unwired: 10 in]
          }
          frame #1 {
            n207 = local write "Load"(FALSE) -> ()
          }
        }
      }
    }
  }
  n208 = local write "Load"(TRUE) -> ()
